vi "Cleanup Device.vi"(8 "error in (no error)":errorcluster, 11 "Simulated PSU in":refnum<class "Simulated PSU.lvclass">) -> (0 "error out":errorcluster, 3 "Simulated PSU out":refnum<class "Simulated PSU.lvclass">)   [LabVIEW 2020, in "Simulated PSU.lvlib" / "Simulated PSU.lvclass"]
uses:
  Simulated PSU.lvclass
  Simulated PSU.lvclass/Simulated PSU.ctl
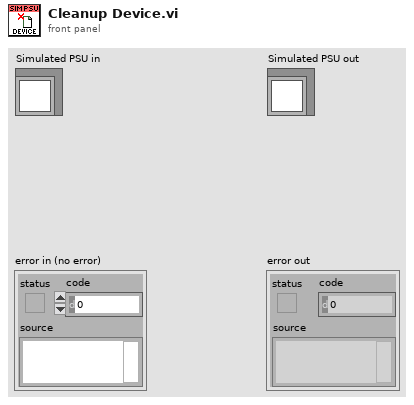
[diagram p1: front panel]
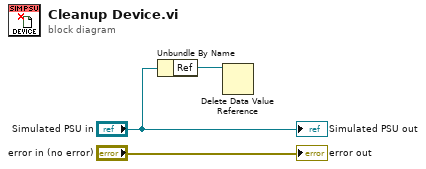
[diagram p0: block diagram]
diagram:
  n1 = Unbundle By Name("Simulated PSU in") -> ("Ref"=w1:refnum<data-value>)
  n2 = Delete Data Value Reference(data value reference=w1) -> ()  [unwired: 1 in, 2 out]
  "error out" <- "error in (no error)"
  "Simulated PSU out" <- "Simulated PSU in"
